vi "Periodic Tasks.vi"(8 "error in":errorcluster) -> ()   [LabVIEW 2016]
doc: "This VI runs in parallel to other tasks. It can contain as many user-defined periodic loops as you need. These can carry out PID or other sorts of timed response."
uses:
  <vilib>/Rock Robotics/WPI/Utilities/WPI_GetSetVariantRefNum.vi
  Robot Global Data.vi
  <vilib>/addons/control/pid/pid.llb/PID (DBL).vi
  <vilib>/Rock Robotics/WPI/RobotDrive/WPI_RobotDriveMecanumDrive_Cartesian.vi
  <vilib>/addons/control/pid/NI_PID_pid.lvlib
panel:
  in  "PID gains":T1={"proportional gain (Kc)"=1.0, "integral time (Ti, min)"=0.01, "derivative time (Td, min)"=0.0} {"derivative time (Td, min)" step=1e-05 format="%.3f"; "integral time (Ti, min)" step=1e-05 format="%.3f"; "proportional gain (Kc)" step=0.05 format="%.3f"}
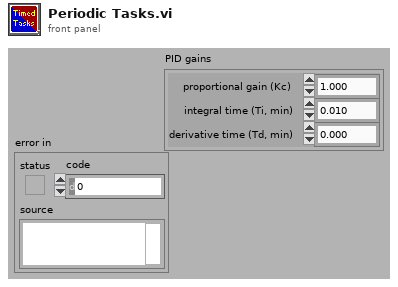
[diagram p1: front panel]
types:
  T1 = cluster{"proportional gain (Kc)":dbl, "integral time (Ti, min)":dbl, "derivative time (Td, min)":dbl}
  T2 = cluster{"Yaw":dbl, "Roll":dbl, "Pitch":dbl, "Heading":dbl, "Fused Heading":dbl}
  T3 = typedef "WPI_JoystickDevRef.ctl" = cluster{"Device":T4}
  T4 = typedef "WPI_JoystickDeviceEnum.ctl" = enum16{"USB 0", "USB 1", "USB 2", "USB 3", "USB 4", "USB 5"}
  T5 = typedef "WPI_RobotDriveDevRef.ctl" = cluster{"DevStatus":errorcluster, "Motors[]":T6[], "Square Inputs":bool, "Max Output":dbl}
  T6 = typedef "WPI_MotorControlDeviceRef.ctl" = cluster{"DeviceStatus":errorcluster, "Type":T7, "PWM":cluster{"PWM Channel":T8, "DeadBand":T9}, "CAN":cluster{"Device Number":u8, "SetOutput VI Ref":variant, "GetOutput VI Ref":variant, "Enable VI Ref":variant, "Disable VI Ref":variant, "Data":variant}, "Invert":bool}
  T7 = typedef "WPI_MotorControlType.ctl" = enum16{"PWM", "CAN"}
  T8 = typedef "FPGA_DIOPWMChannel.ctl" = enum8{"PWM 0", "PWM 1", "PWM 2", "PWM 3", "PWM 4", "PWM 5", "PWM 6", "PWM 7", "PWM 8", "PWM 9", "PWM MXP 0", "PWM MXP 1", "PWM MXP 2", "PWM MXP 3", "PWM MXP 4", "PWM MXP 5", "PWM MXP 6", "PWM MXP 7", "PWM MXP 8", "PWM MXP 9", "Invalid"}
  T9 = typedef "WPI_PWMDeadband.ctl" = cluster{"Name":string, "maxPositivePwm":i32, "minPositivePwm":i32, "centerPwm":i32, "maxNegativePwm":i32, "minNegativePwm":i32, "angularRange":u16}
  T10 = cluster{"JoystickDevRef":T3, "RobotDriveDevRef":T5}
  T11 = typedef "WPI_DriverStationRobotMode2.ctl" = enum16{"Autonomous Disabled", "Autonomous Enabled", "Teleop Disabled", "Teleop Enabled", "Disconnected", "Finish", "Test Disabled", "Test Enabled", "Emergency Stopped"}
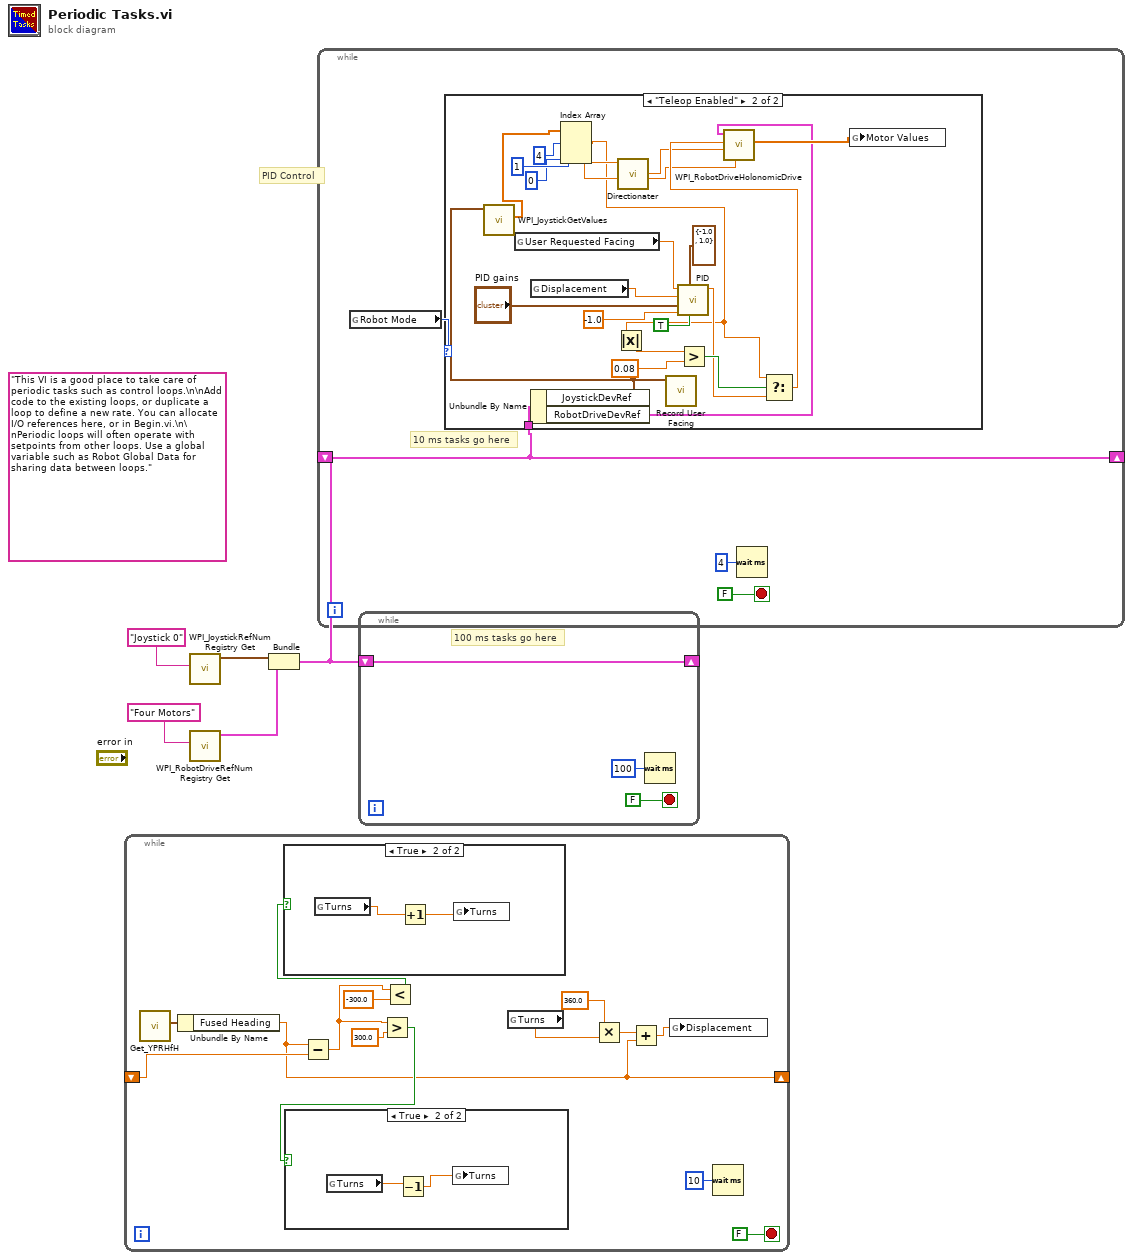
[diagram p0: block diagram]
diagram:
  (unwired) "This VI is a good place to take care of periodic tasks such as control loops.\n\nAdd code to the existing loops, or duplicate a loop to define a new rate. You can allocate I/O references here, or in Begin.vi.\n\nPeriodic loops will often operate with setpoints from other loops. Use a global variable such as Robot Global Data for sharing data between loops."
  # "PID Control"
  n1 = while {
    shift-right: [w11] -> _
    shift-left: _ -> [w17]
    stop <- FALSE stop-if-true
    n2 = call <vilib>:"Get_YPRHfH.vi"() -> ("YRPHfH"=w19:T2)  [unwired: 11 in]
    n3 = Unbundle By Name(w19) -> ("Fused Heading"=w11:dbl)
    n4 = Subtract(x=w11, y=w17) -> (x-y=w7:dbl)
    n5 = Greater?(x=w7, y=300.0 ("x")) -> (0:w15:bool)
    n6 = case shown="True" w15 {
      frame False {
      }
      frame True {
        n7 = global read "Robot Global Data.vi" "Turns"() -> (w20:dbl)
        n8 = Decrement(x=w20) -> (x-1=w21:dbl)
        n9 = global write "Robot Global Data.vi" "Turns"(w21) -> ()
      }
    }
    n10 = Less?(x=w7, y=-300.0) -> (x < y?=w16:bool)
    n11 = case shown="True" w16 {
      frame False {
      }
      frame True {
        n12 = global read "Robot Global Data.vi" "Turns"() -> (w22:dbl)
        n13 = Increment(x=w22) -> (x+1=w23:dbl)
        n14 = global write "Robot Global Data.vi" "Turns"(w23) -> ()
      }
    }
    n15 = global read "Robot Global Data.vi" "Turns"() -> (w13:dbl)
    n16 = Multiply(x=360.0, y=w13) -> (x*y=w12:dbl)
    n17 = Add(x=w12, y=w11) -> (x+y=w10:dbl)
    n18 = global write "Robot Global Data.vi" "Displacement"(w10) -> ()
    n19 = Wait (ms)(milliseconds to wait=u32 10) -> ()  [unwired: 1 out]
  }
  n20 = call <vilib>:"WPI_JoystickRefNum Registry Get.vi"("refnum name"="Joystick 0") -> ("JoystickDevRef"=w3:T3)  [unwired: 1 in, 9 out]
  n21 = call <vilib>:"WPI_RobotDriveRefNum Registry Get.vi"("refnum name"="Four Motors") -> ("RobotDriveDevRef"=w2:T5)  [unwired: 1 in, 9 out]
  n22 = Bundle("JoystickDevRef"=w3, "RobotDriveDevRef"=w2) -> (w1:T10)  [unwired: 1 out]
  n23 = while {
    shift-right: [w24] -> _
    shift-left: w1 -> [w24]
    stop <- FALSE stop-if-true
    # "10 ms tasks go here"
    n24 = global read "Robot Global Data.vi" "Robot Mode"() -> (w25:T11)
    n25 = case shown="\"Teleop Enabled\"" w25 {
      tunnel: w24 -> [_ w51]
      frame "Autonomous Disabled", Default {
      }
      frame "Teleop Enabled" {
        n26 = global read "Robot Global Data.vi" "User Requested Facing"() -> (w40:dbl)
        n27 = global read "Robot Global Data.vi" "Displacement"() -> (w39:dbl)
        n28 = Unbundle By Name(w51) -> ("JoystickDevRef"=w45:T3, "RobotDriveDevRef"=w42:T5)
        n29 = call <vilib>:"WPI_JoystickGetValues.vi"("JoystickDevRef"=w45) -> ("Axes"=w44:dbl[])  [unwired: 6 in, 4 out]
        n30 = Index Array(array=w44, index #1=4 ("index"), index #2=1 ("index"), index #3=0 ("index")) -> (element #1=w30:dbl, element #2=w47:dbl, element #3=w46:dbl)
        n31 = Absolute Value(x=w30) -> (abs(x)=w31:dbl)
        n32 = call "Directionater.vi"("Y In"=w46, "X In"=w47) -> ("Y"=w28:dbl, "Rotation"=w29:dbl)  [unwired: 8 in]
        n33 = call "Record User Facing.vi"("JoystickDevRef"=w45) -> ()  [unwired: 11 in]
        n34 = call-poly <vilib>:"PID.vi"("reinitialize? (F)"=TRUE, "output range"=cluster{"output low":dbl, "output high":dbl} {"output low"=-1.0, "output high"=1.0}, "dt (s)"=-1.0, "PID gains"="PID gains", "process variable"=w39, "setpoint"=w40) -> ("output"=w33:dbl)  [unwired: 4 in, 1 out]
        n35 = Greater?(x=w31, y=0.08 ("x")) -> (0:w34:bool)
        n36 = Select(t=w30, s=w34, f=w33) -> (s? t:f=w32:dbl)
        n37 = call-poly <vilib>:"WPI_RobotDriveHolonomicDrive.vi"("Rotation"=w28, "Y"=w29, "X"=w32, "RobotDriveDevRef"=w42) -> ("Motor Values"=w43:dbl[])  [unwired: 5 in, 2 out]
        n38 = global write "Robot Global Data.vi" "Motor Values"(w43) -> ()
      }
    }
    n39 = Wait (ms)(milliseconds to wait=u32 4) -> ()  [unwired: 1 out]
  }
  n40 = while {
    shift-right: [w52] -> _
    shift-left: w1 -> [w52]
    stop <- FALSE stop-if-true
    # "100 ms tasks go here"
    n41 = Wait (ms)(milliseconds to wait=u32 100) -> ()  [unwired: 1 out]
  }
